vi "SM_Traffic_Lights_main.vi"() -> ()   [LabVIEW 2020]
uses:
  #typedef_Semaphore.ctl
  #typedef_TrafficLights_States.ctl
  #typedef_ProgramData.ctl
  #typedef_Semaphores.ctl
  #typedef_LightTimes.ctl
  #typedef_TimeModes.ctl
  #typedef_TimerAction.ctl
panel:
  in  "Night Mode End":timestamp format="%<%H:%M>T"
  in  "Night Mode Start":timestamp format="%<%H:%M>T"
  in  "stop":bool
  out "West":T1
  out "South":T1
  out "East":T1
  out "North":T1
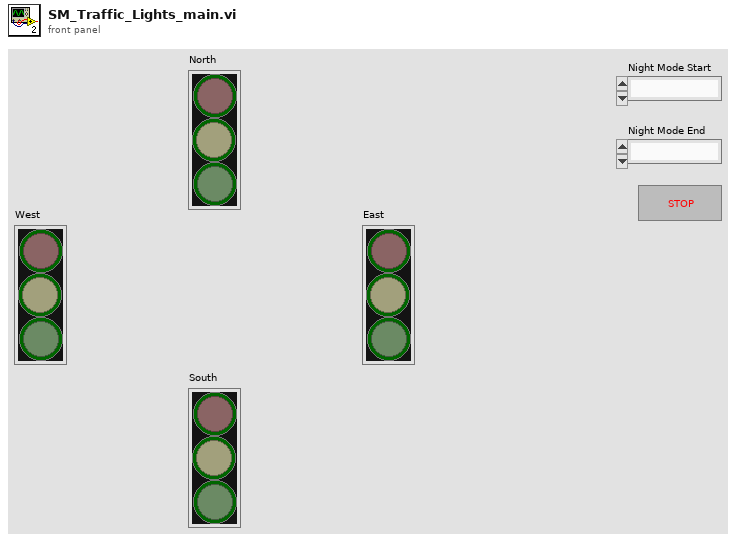
[diagram p1: front panel]
types:
  T1 = typedef "#typedef_Semaphore.ctl" = cluster{"Red":bool, "Yellow":bool, "Green":bool}
  T2 = typedef "#typedef_TrafficLights_States.ctl" = enum16{"Initialize", "Idle", "NS_Green", "NS_Yellow", "NS_Red", "EW_Green", "EW_Yellow", "EW_Red", "NSEW_Yellow_Blink_OFF", "NSEW_Yellow_Blink_ON", "ErrorHandler", "Exit"}
  T3 = typedef "#typedef_TimerAction.ctl" = enum16{"Reset", "TimerElapsed"}
  T4 = typedef "#typedef_ProgramData.ctl" = cluster{"Semaphores":T5, "NextTargetState":T2, "LightTimes":T6, "TimeModes":T7}
  T5 = typedef "#typedef_Semaphores.ctl" = cluster{"North":T1, "East":T1, "South":T1, "West":T1}
  T6 = typedef "#typedef_LightTimes.ctl" = cluster{"Red (2s)":dbl, "Yellow (2s)":dbl, "Green (5s)":dbl, "Blink ON (2s)":dbl, "Blink OFF (2s)":dbl}
  T7 = typedef "#typedef_TimeModes.ctl" = cluster{"Night Mode Start (23:00)":timestamp, "Night Mode End (06:00)":timestamp}
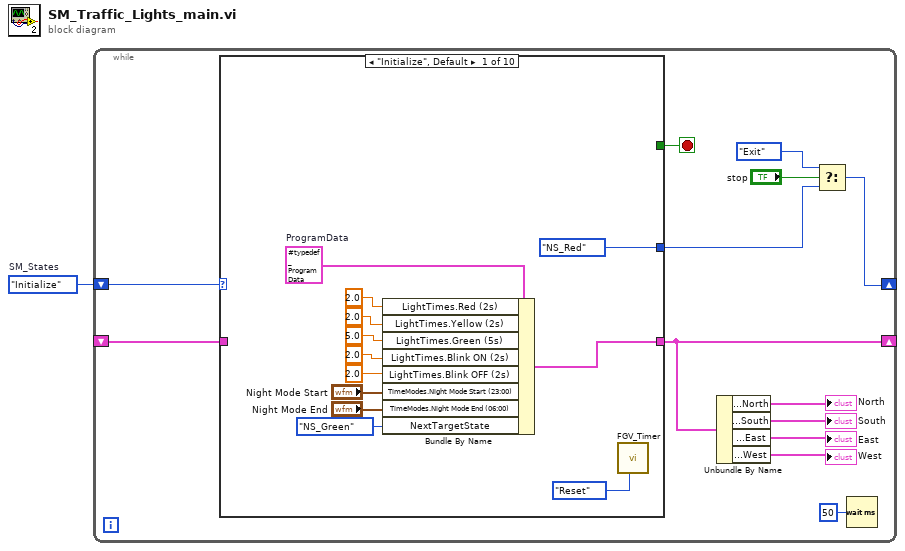
[diagram p0: block diagram]
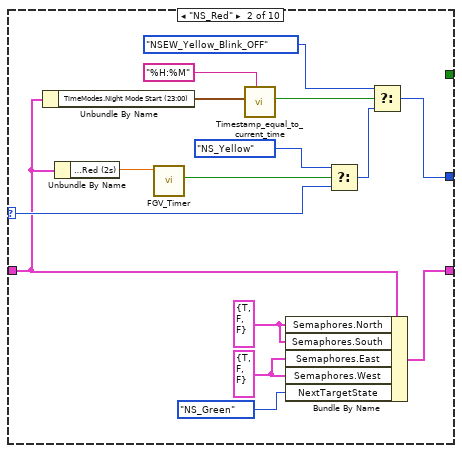
[diagram p2: hidden frame]
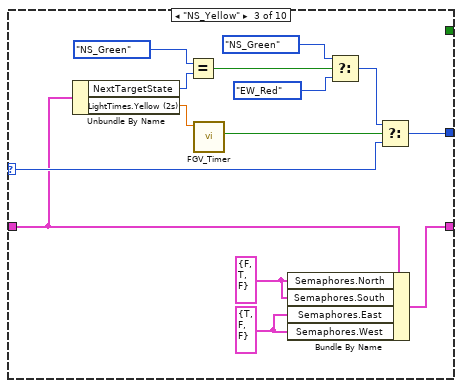
[diagram p3: hidden frame]
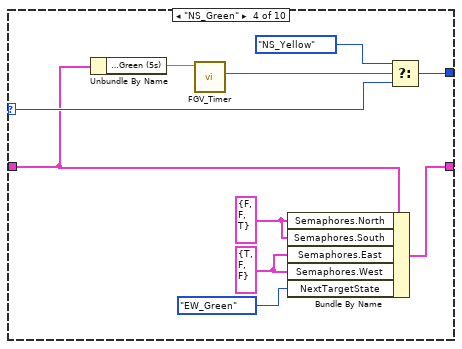
[diagram p4: hidden frame]
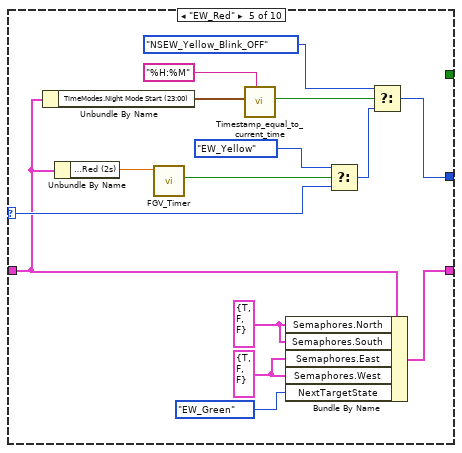
[diagram p5: hidden frame]
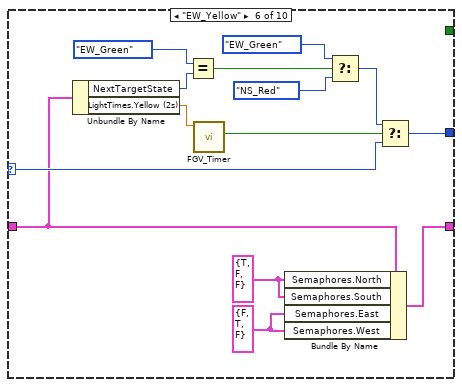
[diagram p6: hidden frame]
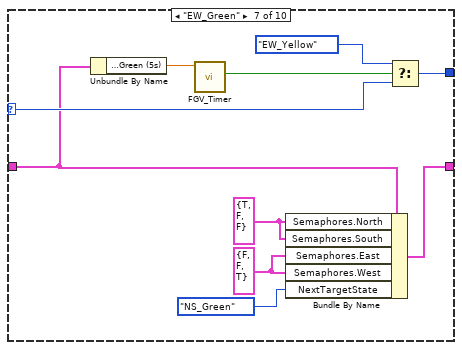
[diagram p7: hidden frame]
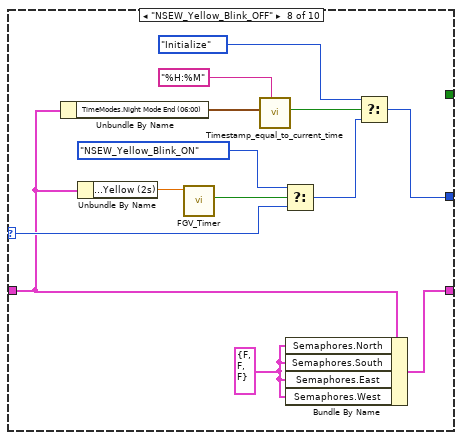
[diagram p8: hidden frame]
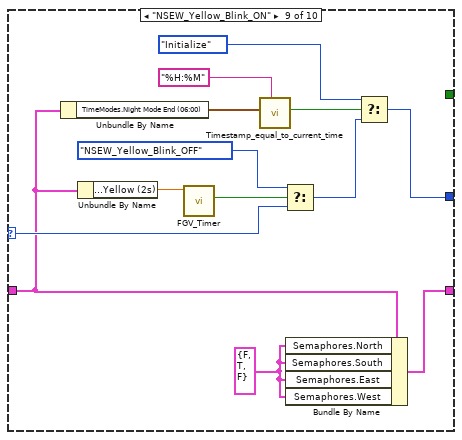
[diagram p9: hidden frame]
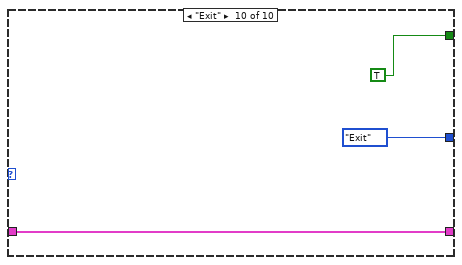
[diagram p10: hidden frame]
diagram:
  w1 = #typedef_TrafficLights_States."Initialize"  # SM_States
  n1 = while {
    shift-right: [w11] -> _
    shift-left: _ -> [w13]
    shift-right: [w3] -> _
    shift-left: w1 -> [w14]
    stop <- w12 stop-if-true
    n2 = case shown="\"Initialize\", Default" w14 {
      selector: w14 -> [_ w39 w47 w64 w78 w86 w103 w116 w129 _]
      tunnel: [w23 w38 w43 w56 w77 w81 w95 w113 w126 w133] -> w11
      tunnel: w13 -> [_ w33 w42 w57 w72 w82 w96 w107 w120 w133]
      tunnel: [#typedef_TrafficLights_States."NS_Red" ("SM_States") w27 w48 w63 w66 w87 w102 w105 w118 #typedef_TrafficLights_States."Exit" ("SM_States")] -> w4
      tunnel: [_ _ _ _ _ _ _ _ _ TRUE] -> w12
      frame "Initialize", Default {
        w24 = T4 {"Semaphores"={"North"={"Red"=TRUE, "Yellow"=FALSE, "Green"=FALSE}, "East"={"Red"=TRUE, "Yellow"=FALSE, "Green"=FALSE}, "South"={"Red"=TRUE, "Yellow"=FALSE, "Green"=FALSE}, "West"={"Red"=TRUE, "Yellow"=FALSE, "Green"=FALSE}}, "NextTargetState"=enum."Initialize", "LightTimes"={"Red (2s)"=2.0, "Yellow (2s)"=2.0, "Green (5s)"=5.0, "Blink ON (2s)"=2.0, "Blink OFF (2s)"=2.0}, "TimeModes"={"Night Mode Start (23:00)"=timestamp(0 s since 1904-01-01), "Night Mode End (06:00)"=timestamp(0 s since 1904-01-01)}}  # ProgramData
        n3 = Bundle By Name(cluster=w24, "LightTimes.Red (2s)"=2.0, "LightTimes.Yellow (2s)"=2.0, "LightTimes.Green (5s)"=5.0, "LightTimes.Blink ON (2s)"=2.0, "LightTimes.Blink OFF (2s)"=2.0, "TimeModes.Night Mode Start (23:00)"="Night Mode Start", "TimeModes.Night Mode End (06:00)"="Night Mode End", "NextTargetState"=#typedef_TrafficLights_States."NS_Green") -> (w23:T4)
        n4 = call "FGV_Timer.vi"("TimerAction (TimerElapsed)"=#typedef_TimerAction."Reset") -> ()  [unwired: 8 in, 3 out]
      }
      frame "NS_Red" {
        w34 = T1 {"Red"=TRUE, "Yellow"=FALSE, "Green"=FALSE} ("Semaphores.North")
        w41 = T1 {"Red"=TRUE, "Yellow"=FALSE, "Green"=FALSE} ("Semaphores.North")
        n5 = Unbundle By Name(w33) -> ("TimeModes.Night Mode Start (23:00)"=w32:timestamp)
        n6 = Unbundle By Name(w33) -> ("LightTimes.Red (2s)"=w37:dbl)
        n7 = call "FGV_Timer.vi"("TimeToElapse (10) (s)"=w37) -> ("Time Elapsed?"=w40:bool)  [unwired: 8 in, 2 out]
        n8 = call "Timestamp_equal_to_current_time.vi"("time format string (%c)"="%H:%M", "time stamp"=w32) -> ("Boolean"=w30:bool)  [unwired: 8 in, 1 out]
        n9 = Bundle By Name(cluster=w33, "Semaphores.North"=w34, "Semaphores.South"=w34, "Semaphores.East"=w41, "Semaphores.West"=w41, "NextTargetState"=#typedef_TrafficLights_States."NS_Green") -> (w38:T4)
        n10 = Select(t=#typedef_TrafficLights_States."NS_Yellow" ("SM_States"), s=w40, f=w39) -> (s? t:f=w28:T2)
        n11 = Select(t=#typedef_TrafficLights_States."NSEW_Yellow_Blink_OFF" ("SM_States"), s=w30, f=w28) -> (s? t:f=w27:T2)
      }
      frame "NS_Yellow" {
        w44 = T1 {"Red"=FALSE, "Yellow"=TRUE, "Green"=FALSE} ("Semaphores.North")
        w45 = T1 {"Red"=TRUE, "Yellow"=FALSE, "Green"=FALSE} ("Semaphores.North")
        n12 = Unbundle By Name(w42) -> ("NextTargetState"=w53:T2, "LightTimes.Yellow (2s)"=w46:dbl)
        n13 = Equal?(x=#typedef_TrafficLights_States."NS_Green" ("SM_States"), y=w53) -> (x = y?=w52:bool)
        n14 = call "FGV_Timer.vi"("TimeToElapse (10) (s)"=w46) -> ("Time Elapsed?"=w50:bool)  [unwired: 8 in, 2 out]
        n15 = Bundle By Name(cluster=w42, "Semaphores.North"=w44, "Semaphores.South"=w44, "Semaphores.East"=w45, "Semaphores.West"=w45) -> (w43:T4)
        n16 = Select(t=#typedef_TrafficLights_States."NS_Green" ("SM_States"), s=w52, f=#typedef_TrafficLights_States."EW_Red" ("SM_States")) -> (s? t:f=w49:T2)
        n17 = Select(t=w49, s=w50, f=w47) -> (s? t:f=w48:T2)
      }
      frame "NS_Green" {
        w58 = T1 {"Red"=FALSE, "Yellow"=FALSE, "Green"=TRUE} ("Semaphores.North")
        w60 = T1 {"Red"=TRUE, "Yellow"=FALSE, "Green"=FALSE} ("Semaphores.North")
        n18 = Unbundle By Name(w57) -> ("LightTimes.Green (5s)"=w62:dbl)
        n19 = call "FGV_Timer.vi"("TimeToElapse (10) (s)"=w62) -> ("Time Elapsed?"=w65:bool)  [unwired: 8 in, 2 out]
        n20 = Bundle By Name(cluster=w57, "Semaphores.North"=w58, "Semaphores.South"=w58, "Semaphores.East"=w60, "Semaphores.West"=w60, "NextTargetState"=#typedef_TrafficLights_States."EW_Green") -> (w56:T4)
        n21 = Select(t=#typedef_TrafficLights_States."NS_Yellow" ("SM_States"), s=w65, f=w64) -> (s? t:f=w63:T2)
      }
      frame "EW_Red" {
        w73 = T1 {"Red"=TRUE, "Yellow"=FALSE, "Green"=FALSE} ("Semaphores.North")
        w80 = T1 {"Red"=TRUE, "Yellow"=FALSE, "Green"=FALSE} ("Semaphores.North")
        n22 = Unbundle By Name(w72) -> ("TimeModes.Night Mode Start (23:00)"=w71:timestamp)
        n23 = Unbundle By Name(w72) -> ("LightTimes.Red (2s)"=w76:dbl)
        n24 = call "FGV_Timer.vi"("TimeToElapse (10) (s)"=w76) -> ("Time Elapsed?"=w79:bool)  [unwired: 8 in, 2 out]
        n25 = call "Timestamp_equal_to_current_time.vi"("time format string (%c)"="%H:%M", "time stamp"=w71) -> ("Boolean"=w69:bool)  [unwired: 8 in, 1 out]
        n26 = Bundle By Name(cluster=w72, "Semaphores.North"=w73, "Semaphores.South"=w73, "Semaphores.East"=w80, "Semaphores.West"=w80, "NextTargetState"=#typedef_TrafficLights_States."EW_Green") -> (w77:T4)
        n27 = Select(t=#typedef_TrafficLights_States."EW_Yellow" ("SM_States"), s=w79, f=w78) -> (s? t:f=w67:T2)
        n28 = Select(t=#typedef_TrafficLights_States."NSEW_Yellow_Blink_OFF" ("SM_States"), s=w69, f=w67) -> (s? t:f=w66:T2)
      }
      frame "EW_Yellow" {
        w83 = T1 {"Red"=TRUE, "Yellow"=FALSE, "Green"=FALSE} ("Semaphores.North")
        w84 = T1 {"Red"=FALSE, "Yellow"=TRUE, "Green"=FALSE} ("Semaphores.North")
        n29 = Unbundle By Name(w82) -> ("NextTargetState"=w92:T2, "LightTimes.Yellow (2s)"=w85:dbl)
        n30 = Equal?(x=#typedef_TrafficLights_States."EW_Green" ("SM_States"), y=w92) -> (x = y?=w91:bool)
        n31 = call "FGV_Timer.vi"("TimeToElapse (10) (s)"=w85) -> ("Time Elapsed?"=w89:bool)  [unwired: 8 in, 2 out]
        n32 = Bundle By Name(cluster=w82, "Semaphores.North"=w83, "Semaphores.South"=w83, "Semaphores.East"=w84, "Semaphores.West"=w84) -> (w81:T4)
        n33 = Select(t=#typedef_TrafficLights_States."EW_Green" ("SM_States"), s=w91, f=#typedef_TrafficLights_States."NS_Red" ("SM_States")) -> (s? t:f=w88:T2)
        n34 = Select(t=w88, s=w89, f=w86) -> (s? t:f=w87:T2)
      }
      frame "EW_Green" {
        w97 = T1 {"Red"=TRUE, "Yellow"=FALSE, "Green"=FALSE} ("Semaphores.North")
        w99 = T1 {"Red"=FALSE, "Yellow"=FALSE, "Green"=TRUE} ("Semaphores.North")
        n35 = Unbundle By Name(w96) -> ("LightTimes.Green (5s)"=w101:dbl)
        n36 = call "FGV_Timer.vi"("TimeToElapse (10) (s)"=w101) -> ("Time Elapsed?"=w104:bool)  [unwired: 8 in, 2 out]
        n37 = Bundle By Name(cluster=w96, "Semaphores.North"=w97, "Semaphores.South"=w97, "Semaphores.East"=w99, "Semaphores.West"=w99, "NextTargetState"=#typedef_TrafficLights_States."NS_Green") -> (w95:T4)
        n38 = Select(t=#typedef_TrafficLights_States."EW_Yellow" ("SM_States"), s=w104, f=w103) -> (s? t:f=w102:T2)
      }
      frame "NSEW_Yellow_Blink_OFF" {
        w112 = T1 {"Red"=FALSE, "Yellow"=FALSE, "Green"=FALSE} ("Semaphores.North")
        n39 = Unbundle By Name(w107) -> ("TimeModes.Night Mode End (06:00)"=w111:timestamp)
        n40 = Unbundle By Name(w107) -> ("LightTimes.Yellow (2s)"=w115:dbl)
        n41 = call "FGV_Timer.vi"("TimeToElapse (10) (s)"=w115) -> ("Time Elapsed?"=w117:bool)  [unwired: 8 in, 2 out]
        n42 = call "Timestamp_equal_to_current_time.vi"("time format string (%c)"="%H:%M", "time stamp"=w111) -> ("Boolean"=w109:bool)  [unwired: 8 in, 1 out]
        n43 = Select(t=#typedef_TrafficLights_States."NSEW_Yellow_Blink_ON" ("SM_States"), s=w117, f=w116) -> (s? t:f=w106:T2)
        n44 = Bundle By Name(cluster=w107, "Semaphores.North"=w112, "Semaphores.South"=w112, "Semaphores.East"=w112, "Semaphores.West"=w112) -> (w113:T4)
        n45 = Select(t=#typedef_TrafficLights_States."Initialize" ("SM_States"), s=w109, f=w106) -> (s? t:f=w105:T2)
      }
      frame "NSEW_Yellow_Blink_ON" {
        w125 = T1 {"Red"=FALSE, "Yellow"=TRUE, "Green"=FALSE} ("Semaphores.North")
        n46 = Unbundle By Name(w120) -> ("TimeModes.Night Mode End (06:00)"=w124:timestamp)
        n47 = Unbundle By Name(w120) -> ("LightTimes.Yellow (2s)"=w128:dbl)
        n48 = call "FGV_Timer.vi"("TimeToElapse (10) (s)"=w128) -> ("Time Elapsed?"=w130:bool)  [unwired: 8 in, 2 out]
        n49 = call "Timestamp_equal_to_current_time.vi"("time format string (%c)"="%H:%M", "time stamp"=w124) -> ("Boolean"=w122:bool)  [unwired: 8 in, 1 out]
        n50 = Select(t=#typedef_TrafficLights_States."NSEW_Yellow_Blink_OFF" ("SM_States"), s=w130, f=w129) -> (s? t:f=w119:T2)
        n51 = Bundle By Name(cluster=w120, "Semaphores.North"=w125, "Semaphores.South"=w125, "Semaphores.East"=w125, "Semaphores.West"=w125) -> (w126:T4)
        n52 = Select(t=#typedef_TrafficLights_States."Initialize" ("SM_States"), s=w122, f=w119) -> (s? t:f=w118:T2)
      }
      frame "Exit" {
      }
    }
    n53 = Unbundle By Name(w11) -> ("Semaphores.North"=→"North":T1, "Semaphores.South"=→"South":T1, "Semaphores.East"=→"East":T1, "Semaphores.West"=→"West":T1)
    n54 = Select(t=#typedef_TrafficLights_States."Exit", s="stop", f=w4) -> (s? t:f=w3:T2)
    n55 = Wait (ms)(milliseconds to wait=u32 50) -> ()  [unwired: 1 out]
  }
